vi "Setup.vi"(5 "Protocol selection\n(appended)":T1 {"Mode" items=["Modbus-1", "3"]}, 7 "protocol selection ref":refnum<vi>, 8 "error in (no error)":errorcluster, 9 "search":bool, 10 "Comm master cluster in":T4={"Main event var"=refnum, "VIRef"=refnum, "Data path"=path "", "Reads"=0, "total number of UUT"=0, "FF refnum"={"Handle1"=0, "Handle2"=0}, "FF device id list"=[], "MODBUS resource name"="", "MODBUS Serial Parameters"={"Mode"=enum."RTU", "Default Slave Address"=0, "MODBUS timeout"=0, "Baud Rate"=0, "Parity"=0, "Flow Control"=0}, "Profibus resource name"="", "Profibus Communication ref.:"=0, "HART resource name"="", "HART long addresses (array)"=[], "Comm relay session"="", "Comm UI event"=refnum, "Write Interval (s)"=5.0, "DMM_QUEUE"=refnum, "POWER_QUEUE"=refnum, "\nTHERM_QUEUE"=refnum, "\nCOMM_QUEUE"=refnum, "TIMING_QUEUE"=refnum, "MAIN_QUEUE"=refnum, "Log path"=path ""} {"Write Interval (s)" min=0.1 max=1000.0 step=0.1}, 11 "DeviceNET in":refnum<class "DeviceNET.lvclass">) -> (0 "error out":errorcluster, 3 "DeviceNET out":refnum<class "DeviceNET.lvclass">)   [LabVIEW 2016, in "DeviceNET.lvclass"]
uses:
  DeviceNET.lvclass
  MASTER_OPC.ctl
  Typedef/event var.ctl
  Typedef/Comm ui action type.ctl
  Typedef/Comm_State_enum.ctl
  Typedef/state var.ctl
  Typedef/Array_of_Comm_mode_and_address_types.ctl
  Typedef/Comm_mode_and_address_type.ctl
  Typedef/Comm_mode_type_combo.ctl
  Typedef/Protocol_enum_type.ctl
  DeviceNET.lvclass/DeviceNET.ctl
  Protocol Class/Protocol.lvclass
  <vilib>/DeviceNet/DeviceNetLIB.lvlib
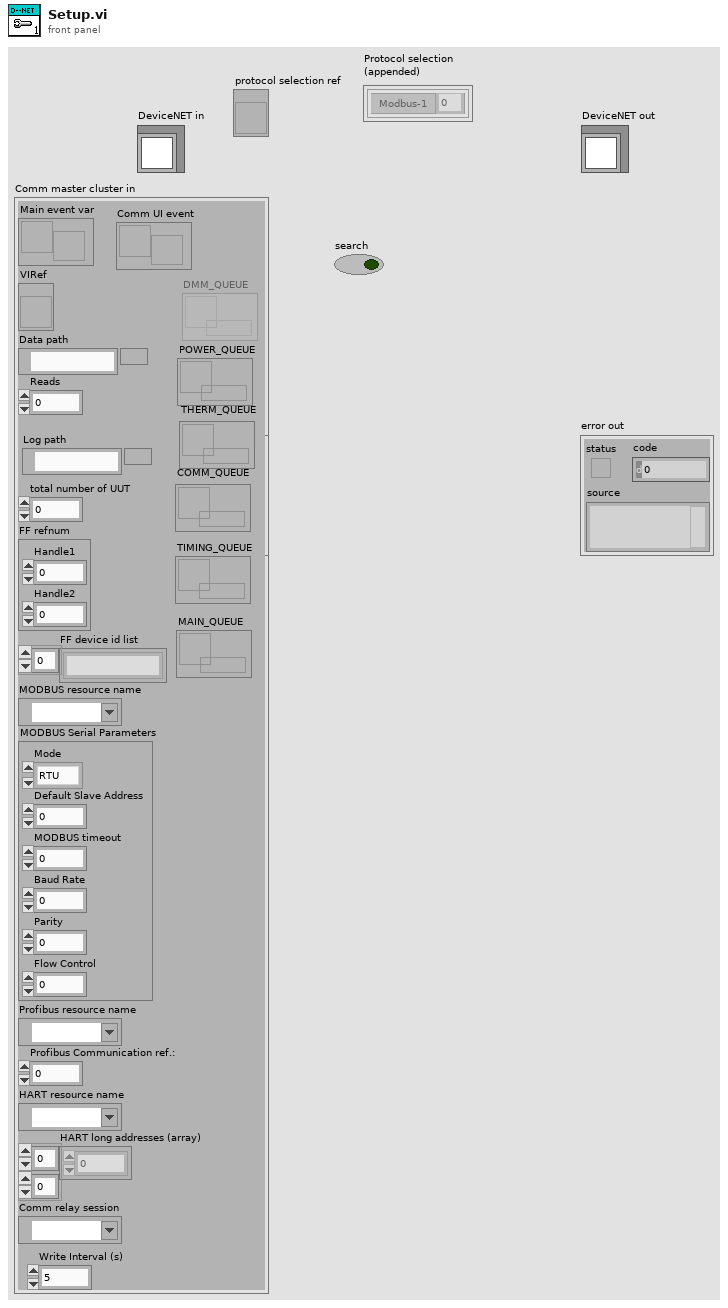
[diagram p1: front panel]
types:
  T1 = typedef "Array_of_Comm_mode_and_address_types.ctl" = T2[]
  T2 = typedef "Comm_mode_and_address_type.ctl" = cluster{"address":i32, "Mode":T3}
  T3 = typedef "Comm_mode_type_combo.ctl" = u16
  T4 = typedef "MASTER_OPC.ctl" = cluster{"Main event var":refnum<user-event>, "VIRef":refnum<vi>, "Data path":path, "Reads":i32, "total number of UUT":i32, "FF refnum":cluster{"Handle1":u32, "Handle2":u32}, "FF device id list":string[], "MODBUS resource name":refnum<visa-resource-name>, "MODBUS Serial Parameters":cluster{"Mode":enum16{"RTU", "ASCII"}, "Default Slave Address":u8, "MODBUS timeout":u32, "Baud Rate":u32, "Parity":u16, "Flow Control":u16}, "Profibus resource name":refnum<visa-resource-name>, "Profibus Communication ref.:":u8, "HART resource name":refnum<visa-resource-name>, "HART long addresses (array)":u8[][], "Comm relay session":refnum<k15>, "Comm UI event":refnum<user-event>, "Write Interval (s)":dbl, "DMM_QUEUE":refnum<queue>, "POWER_QUEUE":refnum<queue>, "\nTHERM_QUEUE":refnum<queue>, "\nCOMM_QUEUE":refnum<queue>, "TIMING_QUEUE":refnum<queue>, "MAIN_QUEUE":refnum<queue>, "Log path":path}
  T5 = typedef "Protocol_enum_type.ctl" = enum16{"None", "MODBUS", "HART", "Fieldbus", "Profibus DP", "Profibus PA", "DeviceNET", "USB"}
  T6 = enum16{"Connect whole bus", "Connect individual UUTs", "Connect none"}
  T7 = cluster{"Device address":i32, "Switch index":i32}
  T8 = cluster{"Device Address":i32, "Switch index":i32}[]
  T9 = cluster{"Device Address":i32, "Switch index":i32}
  T10 = typedef "DeviceNetLIB.lvlib/DnetIntfConfig.ctl" = cluster{"interface MAC ID":u32, "baud rate":enum32{"125000", "250000", "500000"}, "poll mode":enum32{"Automatic", "Scanned", "Individual"}}
  T11 = enum16{"dnet0", "dnet1", "dnet2", "dnet3", "dnet4", "dnet5", "dnet6", "dnet7", "dnet8", "dnet9", "dnet10", "dnet11", "dnet12", "dnet13", "dnet14", "dnet15", "dnet16", "dnet17", "dnet18", "dnet19", "dnet20", "dnet21", "dnet22", "dnet23", "dnet24", "dnet25", "dnet26", "dnet27", "dnet28", "dnet29", "dnet30", "dnet31"}
  T12 = typedef "DeviceNetLIB.lvlib/xobjhandle.ctl" = u32
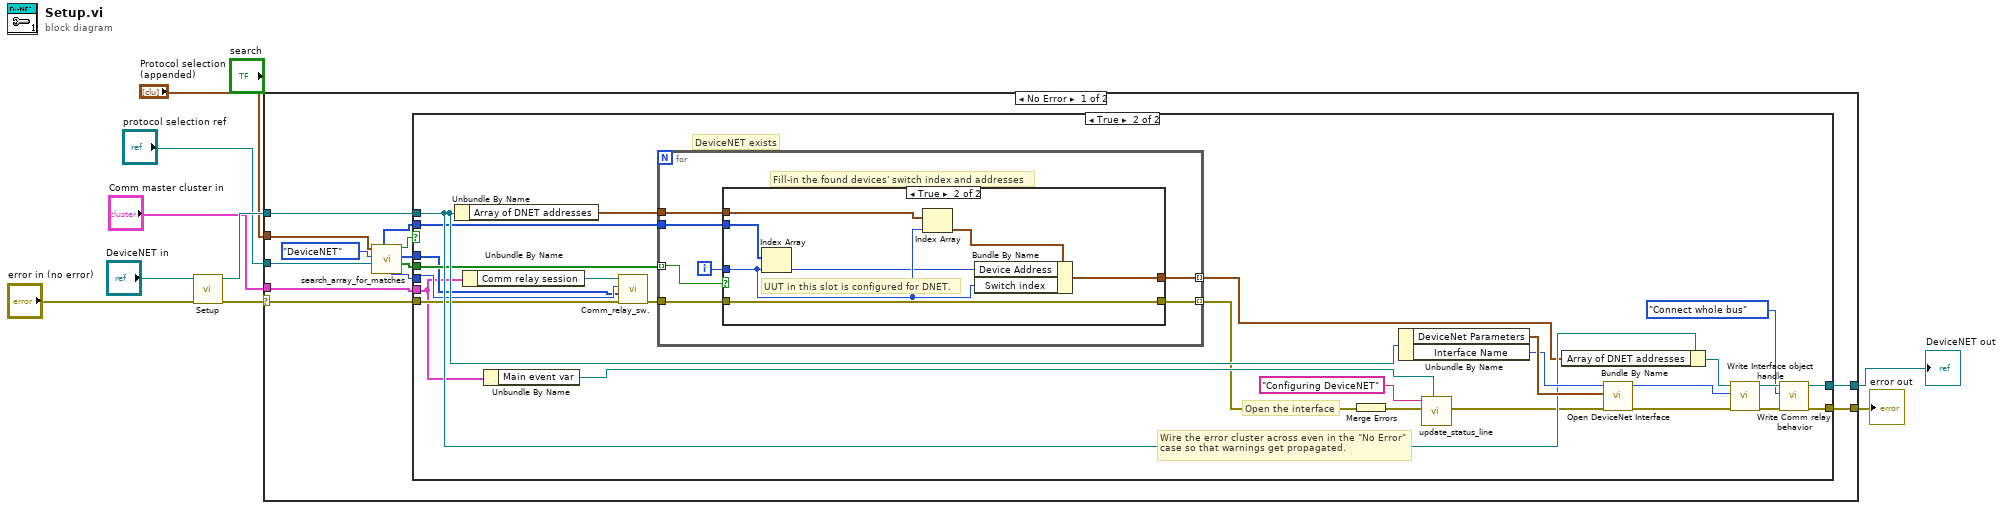
[diagram p0: block diagram]
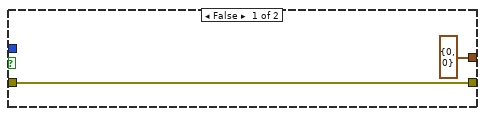
[diagram p3: hidden frame]
diagram:
  n1 = call-parent "Setup.vi"("error in (no error)"="error in (no error)", "Protocol in"="DeviceNET in") -> ("error out"=w7:errorcluster, "Protocol out"=w5:refnum<class "DeviceNET.lvclass">)  [unwired: 8 in]
  n2 = case shown="No Error" w7 {
    selector: w7 -> [w22 w67]
    tunnel: [w19 w67] -> w6
    tunnel: w5 -> [w21 w68]
    tunnel: [w20 w68] -> w4
    tunnel: "Comm master cluster in" -> [w18 _]
    tunnel: "Protocol selection\n(appended)" -> [w16 _]
    tunnel: "protocol selection ref" -> [w14 _]
    frame No Error {
      n3 = call "search_array_for_matches.vi"("protocol selection ref"=w14, "Protocol enum"=Protocol_enum_type."DeviceNET", "appended array"=w16) -> ("Array of exists"=w13:bool[], "array of indexes"=w10:i32[], "exists?"=w15:bool, "Switch Row"=w11:i32, "all addresses"=w12:i32[])  [unwired: 3 in, 1 out]
      n4 = case shown="True" w15 {
        tunnel: w22 -> [w23 w27]
        tunnel: w21 -> [w24 w44]
        tunnel: [w24 w34] -> w20
        tunnel: [w23 w31] -> w19
        tunnel: w18 -> [_ w25]
        tunnel: w12 -> [_ w39]
        tunnel: w13 -> [_ w40]
        tunnel: w11 -> [_ w29]
        tunnel: w10 -> [_ w28]
        frame False {
        }
        frame True {
          # "DeviceNET exists"
          # "Open the interface"
          # "Wire the error cluster across even in the \"No Error\"\ncase so that warnings get propagated."
          n5 = Unbundle By Name(w44) -> ("Array of DNET addresses"=w41:T8)
          n6 = Unbundle By Name(w25) -> ("Comm relay session"=w30:refnum<k15>)
          n7 = Unbundle By Name(w25) -> ("Main event var"=w46:refnum<user-event>)
          n8 = call "Comm_relay_sw..vi"("Error in"=w27, "Columns"=w28, "Row"=w29, "instrument handle in"=w30) -> ("error out"=w26:errorcluster)  [unwired: 6 in, 1 out]
          n9 = for {
            tunnel: w41 -> [w57]
            tunnel: [w56] -> w36 mode=indexing
            tunnel: w26 -> [w55]
            tunnel: [w54] -> w38 mode=indexing
            tunnel: w40 -> [w53] mode=indexing
            tunnel: w39 -> [w51]
            i -> [w52]
            # "Fill-in the found devices' switch index and addresses"
            n10 = case shown="True" w53 {
              tunnel: w57 -> [_ w66]
              tunnel: w51 -> [_ w65]
              tunnel: [T7 {"Device address"=0, "Switch index"=0} ("Hart address") w60] -> w56
              tunnel: w55 -> [w59 w62]
              tunnel: [w59 w62] -> w54
              tunnel: w52 -> [_ w63]
              frame False {
              }
              frame True {
                # "UUT in this slot is configured for DNET."
                n11 = Index Array(array=w65, index=w63) -> (element=w61:i32)
                n12 = Index Array(array=w66, index=w63) -> (element=w64:T9)
                n13 = Bundle By Name(cluster=w64, "Device Address"=w61, "Switch index"=w63) -> (w60:T9)
              }
            }
          }
          n14 = Merge Errors(w38) -> (w37:errorcluster)
          n15 = Unbundle By Name(w44) -> ("DeviceNet Parameters"=w50:T10, "Interface Name"=w49:T11)
          n16 = call "update_status_line.vi"("user event"=w46, "error in (no error)"=w37, "message"="Configuring DeviceNET") -> ("error out"=w42:errorcluster)  [unwired: 7 in, 1 out]
          n17 = Bundle By Name(cluster=w44, "Array of DNET addresses"=w36) -> (w43:refnum<class "DeviceNET.lvclass">)
          n18 = call <vilib>:"Open DeviceNet Interface.vi"("error in (no error)"=w42, "interface configuration"=w50, "interface name"=w49) -> ("error out"=w47:errorcluster, "object handle out"=w48:T12)  [unwired: 3 in]
          n19 = call-dynamic "Write Interface object handle.vi"("error in (no error)"=w47, "ObjHandle"=w48, "DeviceNET in"=w43) -> ("error out"=w32:errorcluster, "DeviceNET out"=w35:refnum<class "DeviceNET.lvclass">)  [unwired: 7 in]
          n20 = call-dynamic "Write Comm relay behavior.vi"("error in (no error)"=w32, "Comm relay behavior"=T6."Connect whole bus", "Protocol in"=w35) -> ("error out"=w31:errorcluster, "Protocol out"=w34:refnum<class "DeviceNET.lvclass">)  [unwired: 7 in]
        }
      }
    }
    frame Error {
    }
  }
  "error out" <- w6
  "DeviceNET out" <- w4
